vi "Memory.Array.Set Pointer.vi"(8 "error in (no error)":errorcluster, 10 "Pointer":refnum<class "Memory.Pointer.lvclass">, 11 "Array in":refnum<class "Memory.Array.lvclass">) -> (0 "error out":errorcluster, 3 "Array out":refnum<class "Memory.Array.lvclass">)   [LabVIEW 2016, in "LabVIEW Memory Manager.lvlib" / "Memory.Array.lvclass"]
uses:
  Memory.Array.lvclass
  Pointer/Memory.Pointer.lvclass
  Memory.Array.lvclass/Memory.Array.ctl
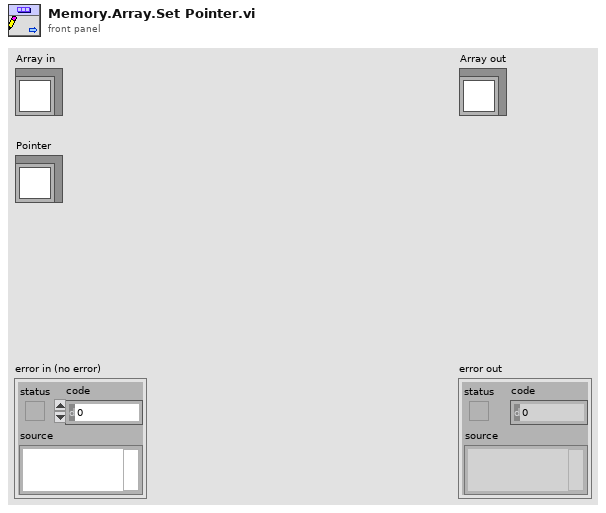
[diagram p1: front panel]
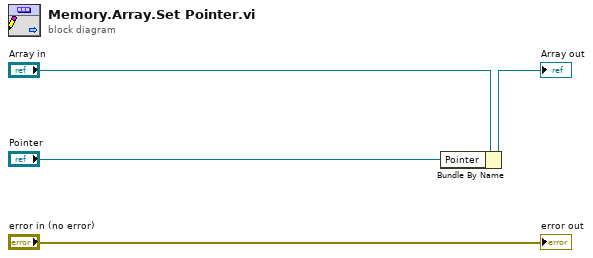
[diagram p0: block diagram]
diagram:
  n1 = Bundle By Name(cluster="Array in", "Pointer"="Pointer") -> (→"Array out":refnum<class "Memory.Array.lvclass">)
  "error out" <- "error in (no error)"
